vi "initialize hardware.vi"(7 "Reset (False)":bool, 8 "error in (no error)":errorcluster, 9 "devport":string, 10 "Settings":T1={"devport"="", "Position"={"Axis 1"={"Value"=0.0, "Min"=0.0, "Max"=0.0, "StepSize"=0.0, "Tolerance"=0.0, "ValueActual"=0.0}, "Axis 2"={"Value"=0.0, "Min"=0.0, "Max"=0.0, "StepSize"=0.0, "Tolerance"=0.0, "ValueActual"=0.0}, "Axis 3"={"Value"=0.0, "Min"=0.0, "Max"=0.0, "StepSize"=0.0, "Tolerance"=0.0, "ValueActual"=0.0}}, "Power"={"Axis 1"=enum."off", "Axis 2"=enum."off", "Axis 3"=enum."off"}, "Status"={"Axis 1"=enum."Not referenced", "Axis 2"=enum."Not referenced", "Axis 3"=enum."Not referenced"}, "Backlash"={"Axis 1"={"Value"=0.0, "Min"=0.0, "Max"=0.0, "StepSize"=0.0, "Tolerance"=0.0, "ValueActual"=0.0}, "Axis 2"={"Value"=0.0, "Min"=0.0, "Max"=0.0, "StepSize"=0.0, "Tolerance"=0.0, "ValueActual"=0.0}, "Axis 3"={"Value"=0.0, "Min"=0.0, "Max"=0.0, "StepSize"=0.0, "Tolerance"=0.0, "ValueActual"=0.0}}, "Home"={"Axis 1"={"Value"=0.0, "Min"=0.0, "Max"=0.0, "StepSize"=0.0, "Tolerance"=0.0, "ValueActual"=0.0}, "Axis 2"={"Value"=0.0, "Min"=0.0, "Max"=0.0, "StepSize"=0.0, "Tolerance"=0.0, "ValueActual"=0.0}, "Axis 3"={"Value"=0.0, "Min"=0.0, "Max"=0.0, "StepSize"=0.0, "Tolerance"=0.0, "ValueActual"=0.0}}, "MoveToHardLimit"={"Axis 1"=enum."pos", "Axis 2"=enum."pos", "Axis 3"=enum."pos"}, "relativeMove"={"Axis 1neg"=enum."off", "Axis 2neg"=enum."off", "Axis 3neg"=enum."off", "Axis 1pos"=enum."off", "Axis 2pos"=enum."off", "Axis 3pos"=enum."off"}, "stepsize"={"Value"=0.0, "Min"=0.0, "Max"=0.0, "StepSize"=0.0, "Tolerance"=0.0, "ValueActual"=0.0}, "automotoroff"=enum."off", "ResetBeforeMove"=enum."off", "Enable"={"Axis 1"=enum."on", "Axis 2"=enum."on", "Axis 3"=enum."on"}, "InitWithDBValues"=enum."off"}, 11 "ESP302 in":refnum<class "ESP302.lvclass">) -> (0 "error out":errorcluster, 2 "VISA resource name out":refnum<visa-resource-name>, 3 "ESP302 out":refnum<class "ESP302.lvclass">)   [LabVIEW 2020, in "ESP302.lvclass"]
uses:
  ESP302.lvclass
  SettingsTypdef.ctl
  OnOffTypeDef.ctl
  status_TypDef.ctl
  Hardware limit.ctl
  ESP302.lvclass/ESP302.ctl
  ESP301.lvclass
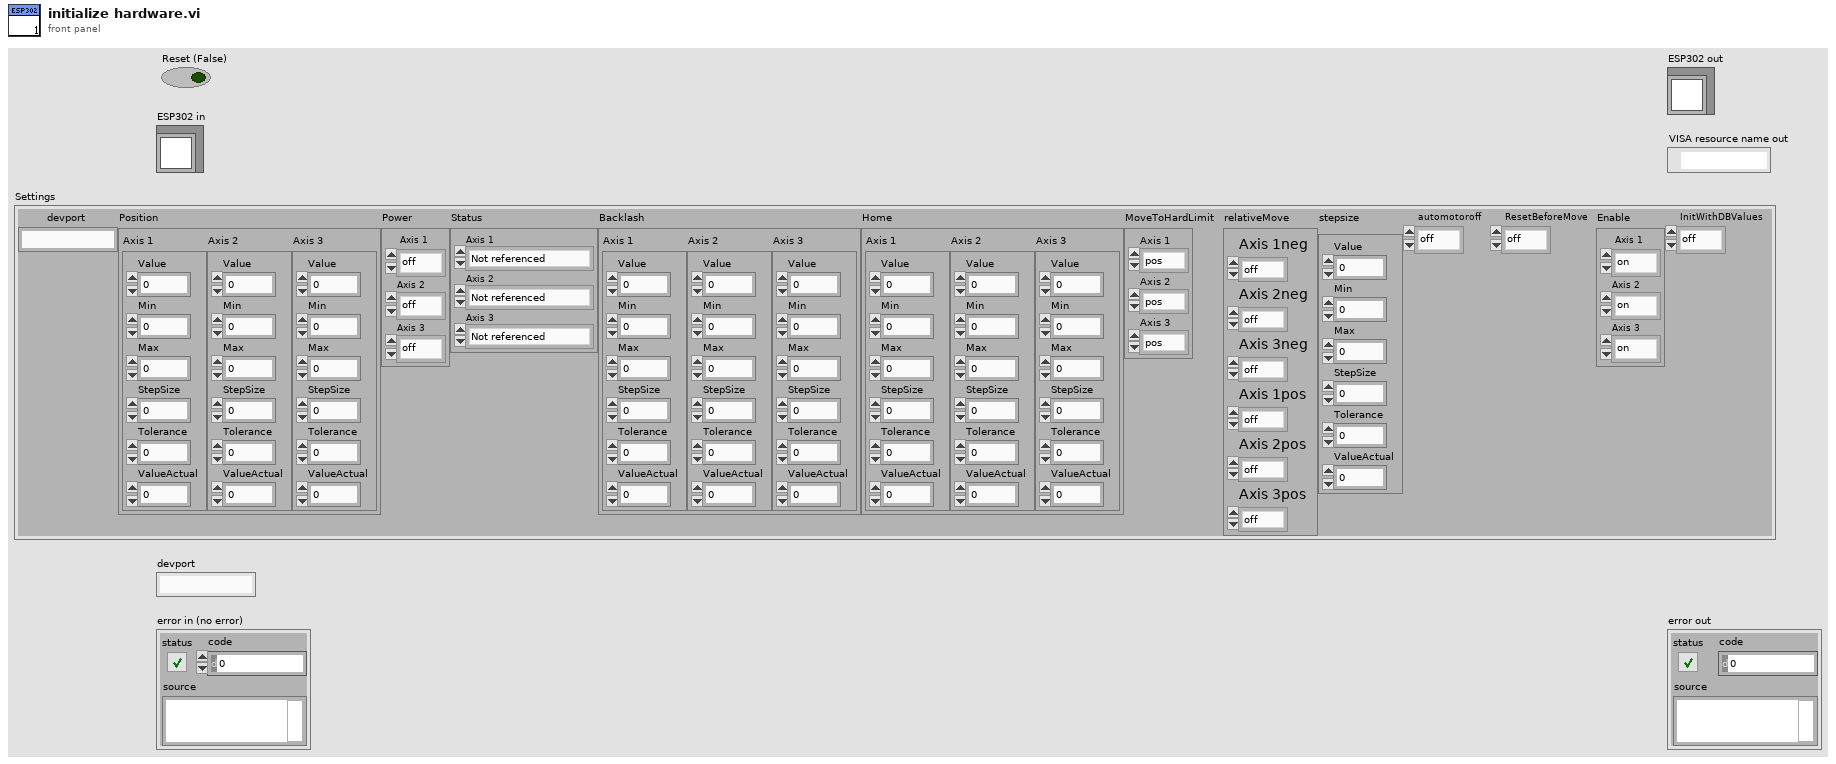
[diagram p1: front panel]
types:
  T1 = typedef "ESP301.lvclass/SettingsTypdef.ctl" = cluster{"devport":string, "Position":cluster{"Axis 1":cluster{"Value":dbl, "Min":dbl, "Max":dbl, "StepSize":dbl, "Tolerance":dbl, "ValueActual":dbl}, "Axis 2":cluster{"Value":dbl, "Min":dbl, "Max":dbl, "StepSize":dbl, "Tolerance":dbl, "ValueActual":dbl}, "Axis 3":cluster{"Value":dbl, "Min":dbl, "Max":dbl, "StepSize":dbl, "Tolerance":dbl, "ValueActual":dbl}}, "Power":cluster{"Axis 1":T2, "Axis 2":T2, "Axis 3":T2}, "Status":cluster{"Axis 1":T3, "Axis 2":T3, "Axis 3":T3}, "Backlash":cluster{"Axis 1":cluster{"Value":dbl, "Min":dbl, "Max":dbl, "StepSize":dbl, "Tolerance":dbl, "ValueActual":dbl}, "Axis 2":cluster{"Value":dbl, "Min":dbl, "Max":dbl, "StepSize":dbl, "Tolerance":dbl, "ValueActual":dbl}, "Axis 3":cluster{"Value":dbl, "Min":dbl, "Max":dbl, "StepSize":dbl, "Tolerance":dbl, "ValueActual":dbl}}, "Home":cluster{"Axis 1":cluster{"Value":dbl, "Min":dbl, "Max":dbl, "StepSize":dbl, "Tolerance":dbl, "ValueActual":dbl}, "Axis 2":cluster{"Value":dbl, "Min":dbl, "Max":dbl, "StepSize":dbl, "Tolerance":dbl, "ValueActual":dbl}, "Axis 3":cluster{"Value":dbl, "Min":dbl, "Max":dbl, "StepSize":dbl, "Tolerance":dbl, "ValueActual":dbl}}, "MoveToHardLimit":cluster{"Axis 1":T4, "Axis 2":T4, "Axis 3":T4}, "relativeMove":cluster{"Axis 1neg":T2, "Axis 2neg":T2, "Axis 3neg":T2, "Axis 1pos":T2, "Axis 2pos":T2, "Axis 3pos":T2}, "stepsize":cluster{"Value":dbl, "Min":dbl, "Max":dbl, "StepSize":dbl, "Tolerance":dbl, "ValueActual":dbl}, "automotoroff":T2, "ResetBeforeMove":T2, "Enable":cluster{"Axis 1":T2, "Axis 2":T2, "Axis 3":T2}, "InitWithDBValues":T2}
  T2 = typedef "OnOffTypeDef.ctl" = enum16{"off", "on"}
  T3 = typedef "status_TypDef.ctl" = enum16{"Not referenced", "Homing", "Moving", "Ready"}
  T4 = typedef "Hardware limit.ctl" = enum16{"pos", "neg"}
  T5 = cluster{"Axis 1":cluster{"Value":dbl, "Min":dbl, "Max":dbl, "StepSize":dbl, "Tolerance":dbl, "ValueActual":dbl}, "Axis 2":cluster{"Value":dbl, "Min":dbl, "Max":dbl, "StepSize":dbl, "Tolerance":dbl, "ValueActual":dbl}, "Axis 3":cluster{"Value":dbl, "Min":dbl, "Max":dbl, "StepSize":dbl, "Tolerance":dbl, "ValueActual":dbl}}
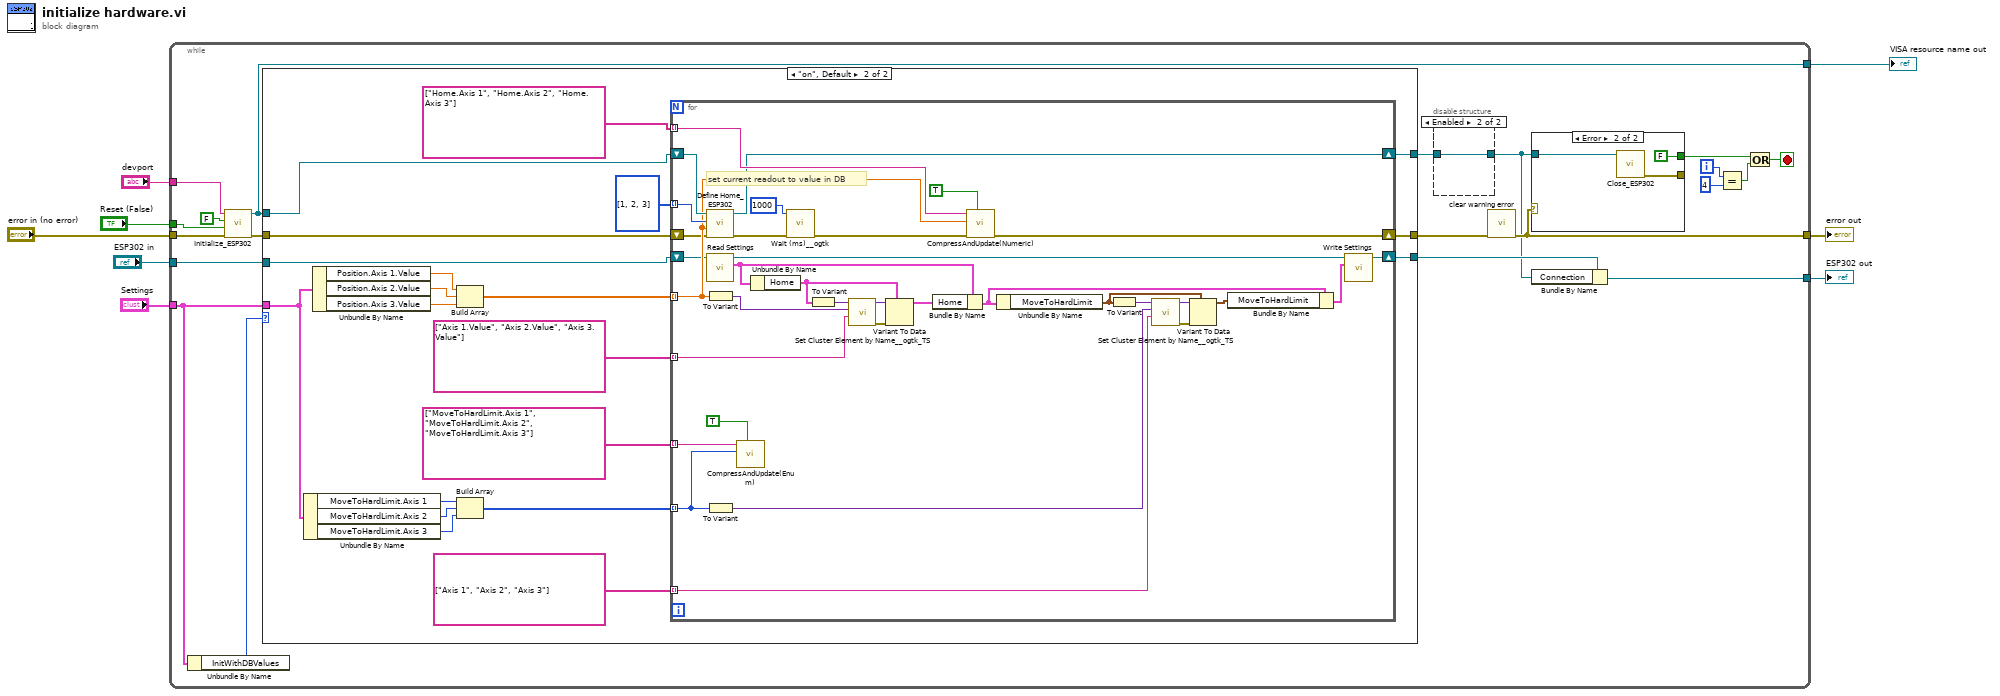
[diagram p0: block diagram]
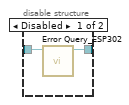
[diagram p3: hidden frame]
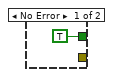
[diagram p4: hidden frame]
diagram:
  n1 = while {
    tunnel: "error in (no error)" -> [w28]
    tunnel: "devport" -> [w26]
    tunnel: "ESP302 in" -> [w14]
    tunnel: [w13] -> w4
    tunnel: [w23] -> w5
    tunnel: "Settings" -> [w10]
    tunnel: [w18] -> w7
    tunnel: "Reset (False)" -> [w15]
    i -> [w22]
    stop <- w19 stop-if-true
    n2 = Unbundle By Name(w10) -> ("InitWithDBValues"=w9:T2)
    n3 = call "Initialize_ESP302.vi"("VISA resource name"=w26, "ID Query (True)"=FALSE, "Reset (False)"=w15, "error in (no error)"=w28) -> ("VISA resource name out"=w23:refnum<visa-resource-name>, "error out"=w16:errorcluster)  [unwired: 5 in]
    n4 = case shown="\"on\", Default" w9 {
      tunnel: [w30 w46] -> w25
      tunnel: [w31 w43] -> w24
      tunnel: w23 -> [w31 w36]
      tunnel: w10 -> [_ w35]
      tunnel: w16 -> [w29 w34]
      tunnel: w14 -> [w30 w33]
      tunnel: [w29 w32] -> w11
      frame "off" {
      }
      frame "on", Default {
        n5 = Unbundle By Name(w35) -> ("MoveToHardLimit.Axis 1"=w39:T4, "MoveToHardLimit.Axis 2"=w40:T4, "MoveToHardLimit.Axis 3"=w41:T4)
        n6 = Unbundle By Name(w35) -> ("Position.Axis 1.Value"=w50:dbl, "Position.Axis 2.Value"=w49:dbl, "Position.Axis 3.Value"=w48:dbl)
        n7 = Build Array(w50, w49, w48) -> (w47:dbl[])
        n8 = Build Array(w39, w40, w41) -> (w38:T4[])
        n9 = for {
          shift-right: [w77] -> w43
          shift-left: w36 -> [w78]
          tunnel: i32[] [1, 2, 3] -> [w76] mode=indexing
          tunnel: w47 -> [w75] mode=indexing
          shift-right: [w55] -> w46
          shift-left: w33 -> [w59]
          tunnel: string[] ["Axis 1.Value", "Axis 2.Value", "Axis 3.Value"] ("set following Variables (empty = all avriables)") -> [w81] mode=indexing
          tunnel: string[] ["Home.Axis 1", "Home.Axis 2", "Home.Axis 3"] ("set following Variables (empty = all avriables)") -> [w79] mode=indexing
          shift-right: [w73] -> w32
          shift-left: w34 -> [w74]
          tunnel: string[] ["MoveToHardLimit.Axis 1", "MoveToHardLimit.Axis 2", "MoveToHardLimit.Axis 3"] ("set following Variables (empty = all avriables)") -> [w71] mode=indexing
          tunnel: w38 -> [w65] mode=indexing
          tunnel: string[] ["Axis 1", "Axis 2", "Axis 3"] ("set following Variables (empty = all avriables)") -> [w64] mode=indexing
          # "set current readout to value in DB"
          n10 = call "Define Home_ESP302.vi"("error in (no error)"=w74, "Home Position (0 units)"=w75, "Axis (1)"=w76, "VISA resource name"=w78) -> ("error out"=w54:errorcluster, "VISA resource name out"=w77:refnum<visa-resource-name>)  [unwired: 2 in]
          n11 = call-dynamic "Read Settings.vi"("ESP301 in"=w59) -> ("Settings"=w58:T1, "ESP301 out"=w57:refnum<class "ESP302.lvclass">)  [unwired: 8 in, 1 out]
          n12 = To Variant(anything=w75) -> (Variant=w61:variant)
          n13 = To Variant(anything=w65) -> (Variant=w62:variant)
          n14 = call "CompressAndUpdate(Enum).vi"("force CVT update (false)"=TRUE ("force CVT update"), "enum variant"=w65, "command or variable name"=w71) -> ()  [unwired: 8 in, 1 out]
          n15 = Unbundle By Name(w58) -> ("Home"=w84:T5)
          n16 = call "Wait (ms)__ogtk.vi"("error in (no error)"=w54, "milliseconds to wait"=u32 1000) -> ("error out"=w53:errorcluster)  [unwired: 8 in, 1 out]
          n17 = To Variant(anything=w84) -> (Variant=w60:variant)
          n18 = call "Set Cluster Element by Name__ogtk_TS.vi"("Element Name (\"\": New Element Data Name)"=w81, "New Element Value"=w61, "Cluster"=w60) -> ("error out"=w82:errorcluster, "VCluster out"=w83:variant)  [unwired: 6 in, 1 out]
          n19 = Variant To Data(error in=w82, type=w84, Variant=w83) -> (data=w85:T5)  [unwired: 1 out]
          n20 = Bundle By Name(cluster=w58, "Home"=w85) -> (w66:T1)
          n21 = call "CompressAndUpdate(Numeric).vi"("force CVT update (false)"=TRUE ("force CVT update"), "error in"=w53, "Numeric"=w75, "command or variable name"=w79) -> ("error out"=w73:errorcluster)  [unwired: 7 in]
          n22 = Unbundle By Name(w66) -> ("MoveToHardLimit"=w68:cluster{"Axis 1":T4, "Axis 2":T4, "Axis 3":T4})
          n23 = To Variant(anything=w68) -> (Variant=w63:variant)
          n24 = call "Set Cluster Element by Name__ogtk_TS.vi"("Element Name (\"\": New Element Data Name)"=w64, "New Element Value"=w62, "Cluster"=w63) -> ("error out"=w70:errorcluster, "VCluster out"=w69:variant)  [unwired: 6 in, 1 out]
          n25 = Variant To Data(error in=w70, type=w68, Variant=w69) -> (data=w67:cluster{"Axis 1":T4, "Axis 2":T4, "Axis 3":T4})  [unwired: 1 out]
          n26 = Bundle By Name(cluster=w66, "MoveToHardLimit"=w67) -> (w56:T1)
          n27 = call-dynamic "Write Settings.vi"("Settings"=w56, "ESP301 in"=w57) -> ("ESP301 out"=w55:refnum<class "ESP302.lvclass">)  [unwired: 8 in, 1 out]
        }
      }
    }
    n28 = disable-structure shown="Enabled" {
      disable-tunnel: w24 -> [w87 w88]
      disable-tunnel: [w86 w88] -> w12
      frame Disabled {
        n29 = call "Error Query_ESP302.vi"("VISA resource name"=w87) -> ("VISA resource name out"=w86:refnum<visa-resource-name>)  [unwired: 3 in, 3 out]
      }
      frame Enabled {
      }
    }
    n30 = call "clear warning error.vi"("error in"=w11) -> ("error out"=w18:errorcluster)  [unwired: 10 in]
    n31 = case shown="Error" w18 {
      tunnel: w12 -> [_ w91]
      tunnel: [TRUE FALSE] -> w17
      tunnel: [_ w90] -> _
      frame No Error {
      }
      frame Error {
        n32 = call "Close_ESP302.vi"("VISA resource name"=w91) -> ("error out"=w90:errorcluster)  [unwired: 10 in]
      }
    }
    n33 = Bundle By Name(cluster=w25, "Connection"=w12) -> (w13:refnum<class "ESP302.lvclass">)
    n34 = Equal?(x=w22, y=4) -> (x = y?=w20:bool)
    n35 = Or(x=w17, y=w20) -> (x .or. y?=w19:bool)
  }
  "error out" <- w7
  "VISA resource name out" <- w5
  "ESP302 out" <- w4
